vi "Write to Table.vi"(8 "Filename":string, 9 "Search For":string, 11 "Input Table":string[][](table)) -> (1 "Found?":bool, 3 "Output Table":string[][](table))   [LabVIEW 2009]
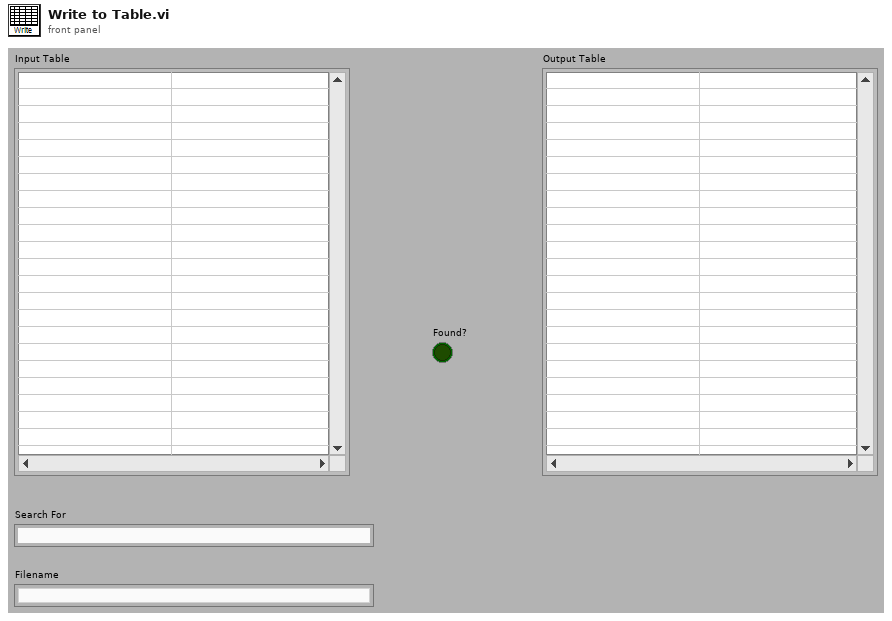
[diagram p1: front panel]
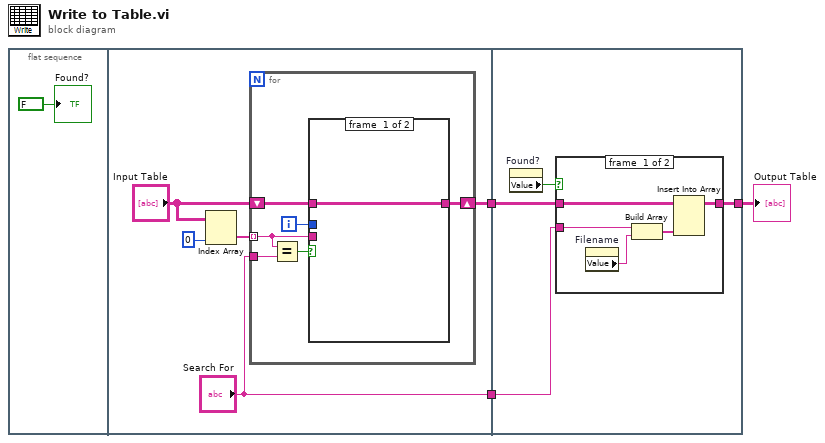
[diagram p0: block diagram]
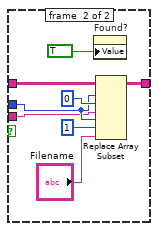
[diagram p2: hidden frame]
diagram:
  n1 = flat-sequence {
    tunnel: [w7] -> w3
    tunnel: ["Search For"] -> w2
    tunnel: w3 -> [w27]
    tunnel: w2 -> [w26]
    tunnel: [w25] -> w1
    frame #0 {
      "Found?" <- FALSE
    }
    frame #1 {
      n2 = Index Array(array="Input Table", index (col)=0) -> (element=w8:string[])  [unwired: 1 in]
      n3 = for {
        tunnel: w8 -> [w13] mode=indexing
        tunnel: "Search For" -> [w15]
        shift-right: [w12] -> w7
        shift-left: "Input Table" -> [w11]
        i -> [w10]
        n4 = Equal?(x=w13, y=w15) -> (x = y?=w14:bool)
        n5 = case shown="True" w14 {
          tunnel: w10 -> [_ w21]
          tunnel: w11 -> [w16 w24]
          tunnel: w13 -> [_ w20]
          tunnel: [w16 w17] -> w12
          frame #0 {
          }
          frame #1 {
            n6 = property on="Found?" class="Bool (strict)"("Value"=TRUE) -> ()  [unwired: 2 in, 2 out]
            n7 = Replace Array Subset(array=w24, new element #1=w20, index (row) #1=w21, index (col) #1=0, new element #2="Filename", index (row) #2=w21, index (col) #2=1) -> (w17:string[][])
          }
        }
      }
    }
    frame #2 {
      n8 = property on="Found?" class="Bool (strict)"() -> ("Value"=w28:bool)  [unwired: 2 in, 2 out]
      n9 = case shown="False" w28 {
        tunnel: w27 -> [w33 w34]
        tunnel: [w29 w34] -> w25
        tunnel: w26 -> [w32 _]
        frame #0 {
          n10 = property on="Filename" class="Str"() -> ("Value"=w31:string)  [unwired: 2 in, 2 out]
          n11 = Build Array(w32, w31) -> (w30:string[])
          n12 = Insert Into Array(array=w33, new element=w30) -> (w29:string[][])  [unwired: 2 in]
        }
        frame #1 {
        }
      }
    }
  }
  "Output Table" <- w1
